vi "isConnected.vi"(8 "error in (no error)":errorcluster, 11 "TCPConnection in":refnum<class "TCPConnection.lvclass">) -> (0 "error out":errorcluster, 2 "connected":bool, 3 "TCPConnection out":refnum<class "TCPConnection.lvclass">)   [LabVIEW 2013]
uses:
  TCPConnection.lvclass
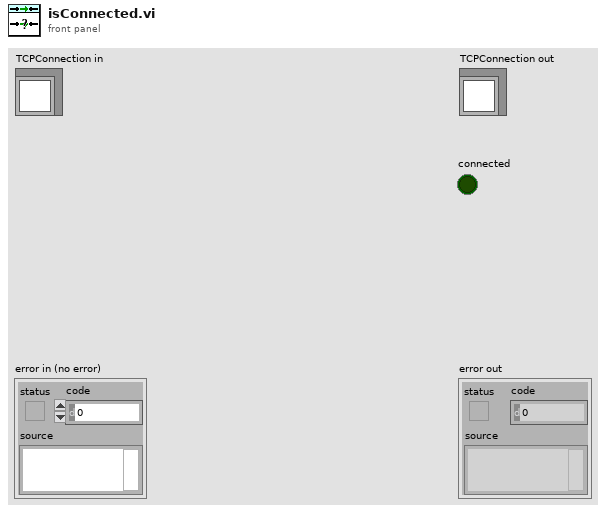
[diagram p1: front panel]
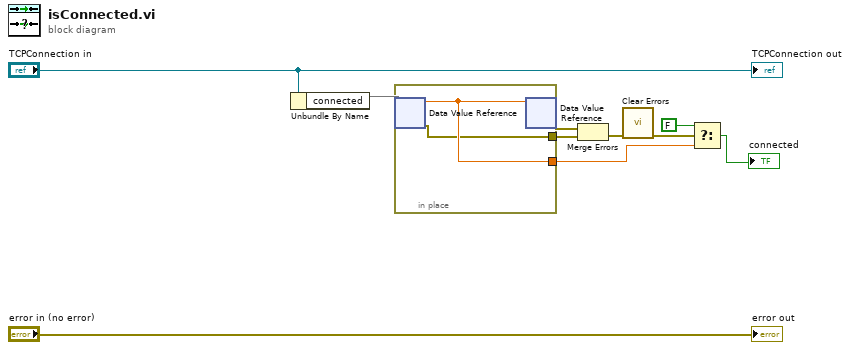
[diagram p0: block diagram]
diagram:
  n1 = Unbundle By Name("TCPConnection in") -> ("connected"=w8)
  n2 = in-place {
    in-place-border: [w12] -> w1
    in-place-border: [w11] -> w6
    n3 = in-place-dvr #1(w8) -> (w12:dbl, w11:errorcluster)
    n4 = in-place-dvr #1(w12) -> (w7:errorcluster)  [unwired: 1 out]
  }
  n5 = Merge Errors(w7, w6) -> (w5:errorcluster)
  n6 = call <vilib>:"Clear Errors.vi"("error in (no error)"=w5) -> ("error out"=w4:errorcluster)  [unwired: 6 in]
  n7 = Select(t=FALSE, s=w4, f=w1) -> (s? t:f=→"connected":bool)
  "error out" <- "error in (no error)"
  "TCPConnection out" <- "TCPConnection in"
